vi "VII Read Bytes.vi"(0 "DevType":i32, 1 "SubAddr":i32, 2 "Len":u16, 5 "DevIndex":i32, 7 "I2CIndex":i32, 9 "SlaveAddr":u16, 11 "error in (no error)":errorcluster, 12 "pReadData":string) -> (4 "function return":i32, 14 "pReadData out":string, 15 "error out":errorcluster)   [LabVIEW 2011, in "ControlI2C.lvlib"]
doc: "int __stdcall VII_ReadBytes(int DevType,int DevIndex,int I2CIndex,unsigned short SlaveAddr,int SubAddr,unsigned char *pReadData,unsigned short Len);"
uses:
  ControlI2C.lvlib
  1234/Ginkgo_Driver.dll
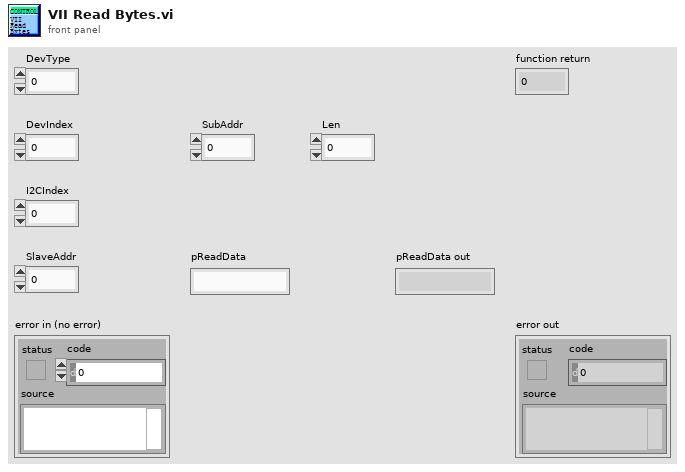
[diagram p1: front panel]
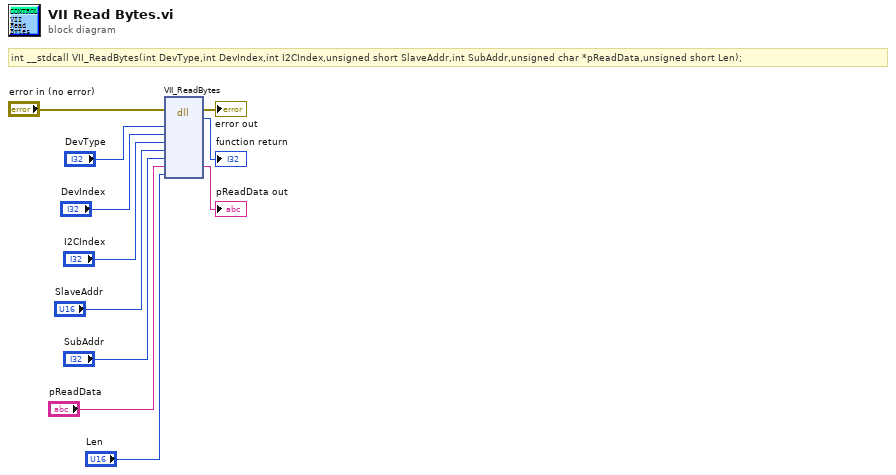
[diagram p0: block diagram]
diagram:
  # "int __stdcall VII_ReadBytes(int DevType,int DevIndex,int I2CIndex,unsigned short SlaveAddr,int SubAddr,unsigned char *pReadData,unsigned short Len);"
  n1 = dll-call lib="E:/Project/vt_ginkgo/truck/Ginkgo Driver/vs2010/Ginkgo_USB-I2C&SPI&CAN_API_v2.0.3.3/lib/labview_32bit/1234/Ginkgo_Driver.*" fn="VII_ReadBytes"(error in="error in (no error)", "DevType"="DevType", "DevIndex"="DevIndex", "I2CIndex"="I2CIndex", "SlaveAddr"="SlaveAddr", "SubAddr"="SubAddr", "pReadData"="pReadData", "Len"="Len") -> (error out=→"error out":errorcluster, →"function return":i32, "pReadData"=→"pReadData out":string)  [unwired: 8 in, 1 out]
